vi "button DIR.vi"(0 "Buttons Control":T2) -> (1 "Direction 2":T1, 2 "LED":bool)   [LabVIEW 2015]
uses:
  Twin Shock/DIR GAME.ctl
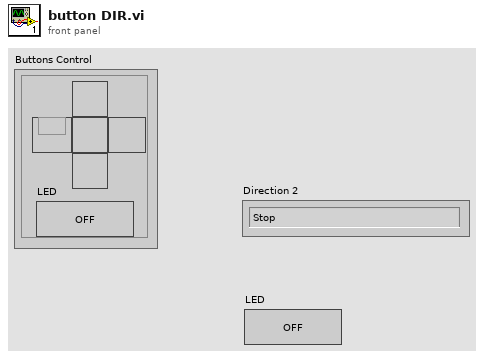
[diagram p1: front panel]
types:
  T1 = typedef "DIR GAME.ctl" = enum16{"Stop", "Front", "FR", "Right", "BR", "Back", "BL", "Left", "FL"}
  T2 = cluster{"Front":bool, "Right":bool, "Back":bool, "Left":bool, "Stop":bool, "LED":bool}
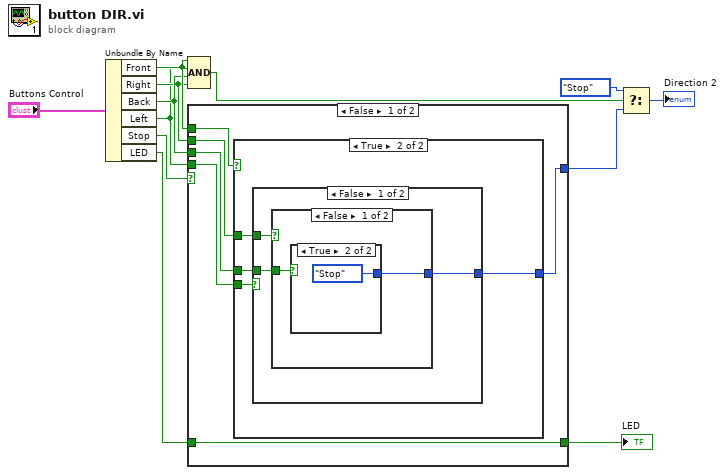
[diagram p0: block diagram]
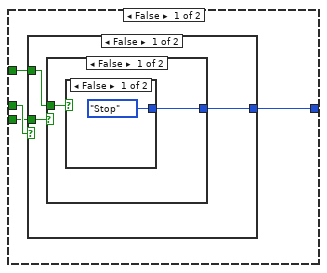
[diagram p2: hidden frame]
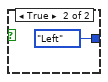
[diagram p3: hidden frame]
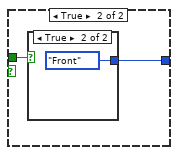
[diagram p4: hidden frame]
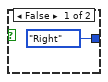
[diagram p5: hidden frame]
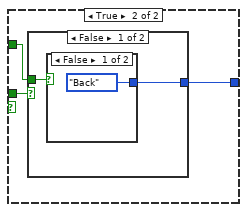
[diagram p6: hidden frame]
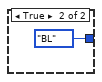
[diagram p7: hidden frame]
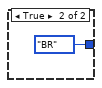
[diagram p8: hidden frame]
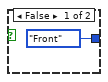
[diagram p9: hidden frame]
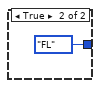
[diagram p10: hidden frame]
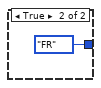
[diagram p11: hidden frame]
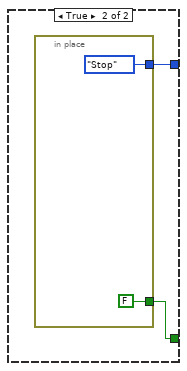
[diagram p12: hidden frame]
diagram:
  n1 = Unbundle By Name("Buttons Control") -> ("Front"=w8:bool, "Right"=w2:bool, "Back"=w7:bool, "Left"=w1:bool, "Stop"=w11:bool, "LED"=w9:bool)
  n2 = Compound Arithmetic op=AND(w8, w1, w7, w2) -> (w3:bool)
  n3 = case shown="False" w11 {
    tunnel: [w15 w56] -> w5
    tunnel: [w18 w55] -> w10
    tunnel: w9 -> [w18 _]
    tunnel: w8 -> [w17 _]
    tunnel: w1 -> [w16 _]
    tunnel: w2 -> [w14 _]
    tunnel: w7 -> [w13 _]
    frame False {
      n4 = case shown="True" w17 {
        tunnel: w16 -> [w21 w45]
        tunnel: [w20 w44] -> w15
        tunnel: w14 -> [w19 w43]
        tunnel: w13 -> [w22 w42]
        frame False {
          n5 = case shown="False" w22 {
            tunnel: w21 -> [w25 w36]
            tunnel: [w23 w35] -> w20
            tunnel: w19 -> [w24 w34]
            frame False {
              n6 = case shown="False" w25 {
                tunnel: w24 -> [w27 w31]
                tunnel: [w26 w30] -> w23
                frame False {
                  n7 = case shown="False" w27 {
                    tunnel: [DIR_GAME."Stop" ("Direction 3") DIR_GAME."Left" ("Direction 3")] -> w26
                    frame False {
                    }
                    frame True {
                    }
                  }
                }
                frame True {
                  n8 = case shown="True" w31 {
                    tunnel: [DIR_GAME."Right" ("Direction 3") DIR_GAME."Front" ("Direction 3")] -> w30
                    frame False {
                    }
                    frame True {
                    }
                  }
                }
              }
            }
            frame True {
              n9 = case shown="False" w36 {
                tunnel: [w37 DIR_GAME."BR" ("Direction 3")] -> w35
                tunnel: w34 -> [w38 _]
                frame False {
                  n10 = case shown="False" w38 {
                    tunnel: [DIR_GAME."Back" ("Direction 3") DIR_GAME."BL" ("Direction 3")] -> w37
                    frame False {
                    }
                    frame True {
                    }
                  }
                }
                frame True {
                }
              }
            }
          }
        }
        frame True {
          n11 = case shown="False" w45 {
            tunnel: [w47 DIR_GAME."FR" ("Direction 3")] -> w44
            tunnel: w43 -> [w48 _]
            tunnel: w42 -> [w46 _]
            frame False {
              n12 = case shown="False" w48 {
                tunnel: [w50 DIR_GAME."FL" ("Direction 3")] -> w47
                tunnel: w46 -> [w49 _]
                frame False {
                  n13 = case shown="True" w49 {
                    tunnel: [DIR_GAME."Front" ("Direction 3") DIR_GAME."Stop" ("Direction 3")] -> w50
                    frame False {
                    }
                    frame True {
                    }
                  }
                }
                frame True {
                }
              }
            }
            frame True {
            }
          }
        }
      }
    }
    frame True {
      n14 = in-place {
        in-place-border: [DIR_GAME."Stop" ("Direction 3")] -> w56
        in-place-border: [FALSE] -> w55
      }
    }
  }
  "LED" <- w10
  n15 = Select(t=DIR_GAME."Stop", s=w3, f=w5) -> (s? t:f=→"Direction 2":T1)
